vi "Get_Calib_zero_Offset.vi"(1 "Measurement Time":dbl format="%#.0f", 2 "Calib Filename":path) -> (0 "Voltage Offset":dbl)   [LabVIEW 2022 SP3]
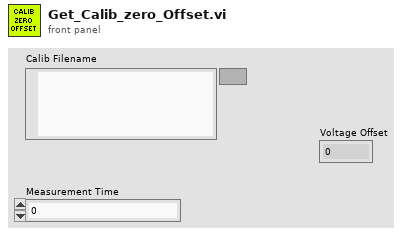
[diagram p1: front panel]
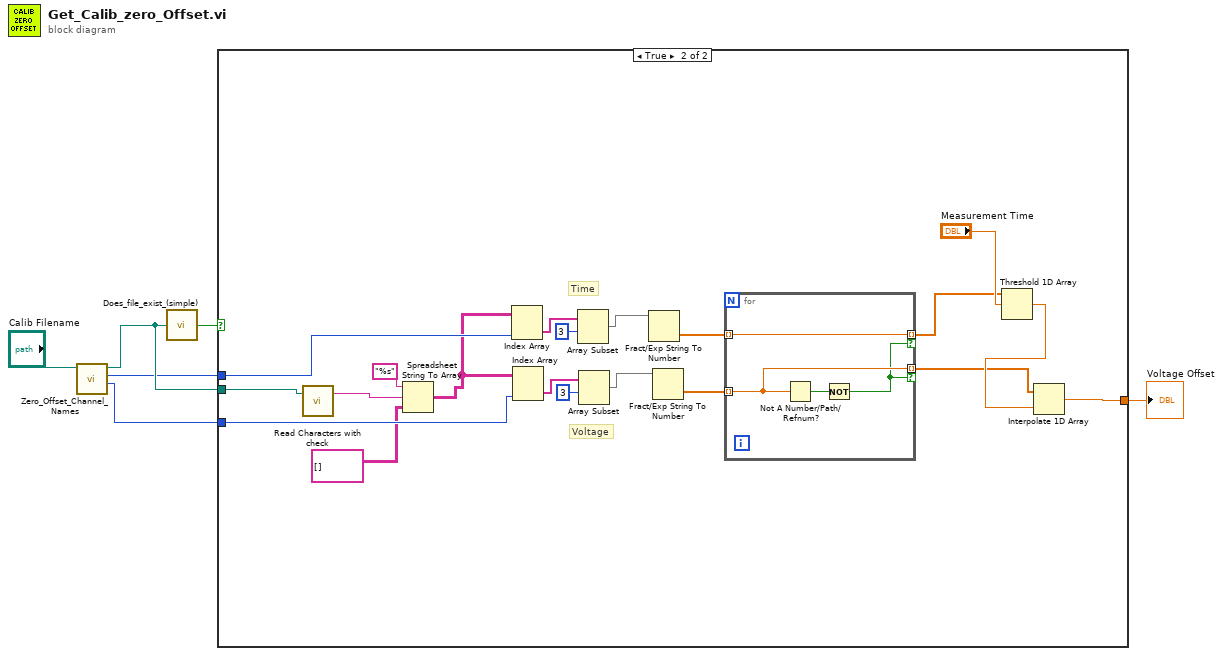
[diagram p0: block diagram]
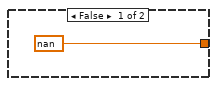
[diagram p2: hidden frame]
diagram:
  n1 = call "Zero_Offset_Channel_Names.vi"("Calib Filename"="Calib Filename") -> ("Voltage Index"=w2:i32, "Time Index"=w3:i32, "Zero Filename"=w4:path)  [unwired: 3 in, 1 out]
  n2 = call "Does_file_exist_(simple).vi"("Pathname"=w4) -> ("exists?"=w5:bool)
  n3 = case shown="True" w5 {
    tunnel: w4 -> [_ w9]
    tunnel: w3 -> [_ w27]
    tunnel: w2 -> [_ w21]
    tunnel: [nan w14] -> w1
    frame False {
    }
    frame True {
      # "Voltage"
      # "Time"
      n4 = call "Read Characters with check.vi"("file (use dialog)"=w9) -> ("Read String"=w8:string)  [unwired: 1 in, 1 out]
      n5 = Spreadsheet String To Array(format string="%s", spreadsheet string=w8, array type (2D Dbl)=string[][] []) -> (array=w22:string[][])  [unwired: 1 in]
      n6 = Index Array(array=w22, index (col)=w27) -> (element=w26:string[])  [unwired: 1 in]
      n7 = Index Array(array=w22, index (col)=w21) -> (element=w23:string[])  [unwired: 1 in]
      n8 = Array Subset(array=w26, index=3) -> (w18:string[])  [unwired: 1 in]
      n9 = Array Subset(array=w23, index=3) -> (w16:string[])  [unwired: 1 in]
      n10 = Fract/Exp String To Number(string=w18) -> (number=w10:dbl[])  [unwired: 3 in, 1 out]
      n11 = Fract/Exp String To Number(string=w16) -> (number=w13:dbl[])  [unwired: 3 in, 1 out]
      n12 = for {
        tunnel: w13 -> [w31] mode=indexing
        tunnel: [w31] -> w12 mode=indexing if=w28
        tunnel: [w29] -> w11 mode=indexing if=w28
        tunnel: w10 -> [w29] mode=indexing
        n13 = Not A Number/Path/Refnum?(number/path/refnum=w31) -> (NaN/Path/Refnum?=w30:bool)
        n14 = Not(x=w30) -> (.not. x?=w28:bool)
      }
      n15 = Threshold 1D Array(2:"Measurement Time", 3:w11) -> (0:w15:dbl)  [unwired: 1 in]
      n16 = Interpolate 1D Array(1:w15, 2:w12) -> (0:w14:dbl)
    }
  }
  "Voltage Offset" <- w1
